vi "Query - DBL - Scalar.vi"(8 "error in":errorcluster, 10 "Query":string, 11 "Module ID":i32=-1) -> (0 "error out":errorcluster, 1 "Meta Data":variant, 2 "Return Data":dbl, 4 "Field Names":string[](array[string]))   [LabVIEW 2020, in "hse-db.lvlib" / "DB_CONNECTOR.lvlib"]
doc: "____\nHAMPEL SOFTWARE ENGINEERING v1.4.0 (2023-12-19 09:52)"
uses:
  DB_CONNECTOR.lvlib
  hse-libraries/Source/hse-misc/Conversion/ConvertStringToFloat_Array-2D.vi
  hse-libraries/Source/hse-misc/hse-misc.lvlib
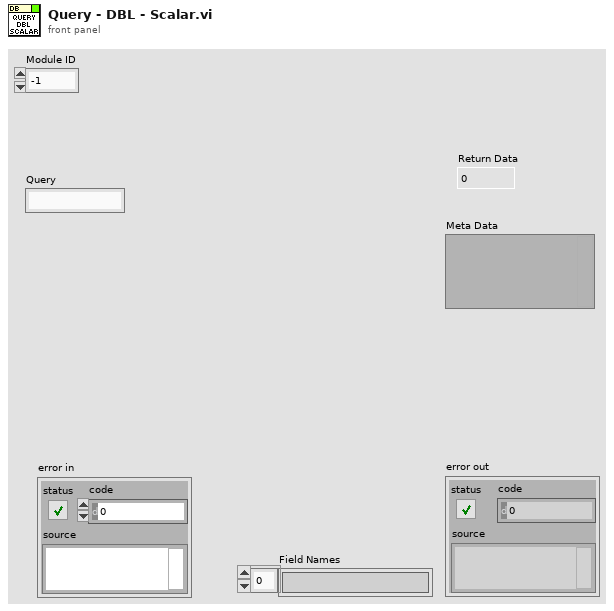
[diagram p1: front panel]
types:
  T1 = typedef "hse-db.lvlib/DB_CONNECTOR.lvlib/Query (Reply Payload)--cluster.ctl" = cluster{"Return Data":string[][], "Meta Data":variant, "Field Names":string[], "Query_error":errorcluster, "Module ID":i32}
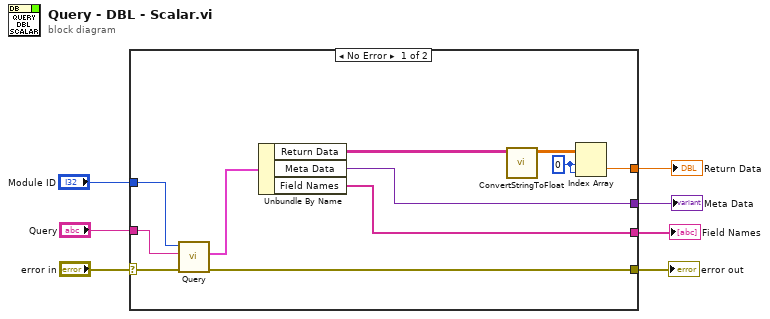
[diagram p0: block diagram]
diagram:
  n1 = case shown="No Error" "error in" {
    selector: "error in" -> [w12 w19]
    tunnel: [w11 w19] -> w6
    tunnel: "Query" -> [w10 _]
    tunnel: "Module ID" -> [w9 _]
    tunnel: [w17 _] -> w2
    tunnel: [w15 _] -> w3
    tunnel: [w13 _] -> w1
    frame No Error {
      w16 = 0 ("index (row)")
      n2 = call "Query.vi"("error in (no error)"=w12, "Query"=w10, "Module ID"=w9) -> ("error out"=w11:errorcluster, "Reply Payload"=w8:T1)  [unwired: 6 in, 1 out]
      n3 = Unbundle By Name(w8) -> ("Return Data"=w18:string[][], "Meta Data"=w17:variant, "Field Names"=w13:string[])
      n4 = call-poly "ConvertStringToFloat.vi"("String"=w18) -> ("Array of Doubles"=w14:dbl[][])  [unwired: 9 in, 1 out]
      n5 = Index Array(array=w14, index (row)=w16, index (col)=w16) -> (element=w15:dbl)
    }
    frame Error {
    }
  }
  "error out" <- w6
  "Return Data" <- w3
  "Meta Data" <- w2
  "Field Names" <- w1
